vi "ExSpecDebugAppCamera.vi"() -> ()   [LabVIEW 2010]
uses:
  GlobalSpectHdl.vi
  GlobalCamHandle.vi
  GlobalCamOpen.vi
  GlobalInitializeFlag.vi
  GlobalFramesToStr.vi
  GlobalTimingMode.vi
  GlobalAcquireFocusFlag.vi
  GlobalExposure.vi
  GlobalUserBin.vi
  GlobalCenter.vi
  GlobalFullBin.vi
  GlobalReverseFlag.vi
  GlobalIBackImgHndl.vi
  GlobalIFlatImgHndl.vi
panel:
  out "Spectrometer\n active":bool
  out "Camera Opened":bool
  in  "Exit program":bool
  out "error out":errorcluster
  in  "error in (no error)":errorcluster
  in  "Tab Control":T1(tab)
  in  "Focus/Acquire Mode":u32=1 min=1 max=5 step=1
  in  "Number of Frames to store":u32=1 min=1 step=1
  in  "Intensifier":bool
  in  "Readout Port":i32=-1 min=-1 step=1
  in  "ADC Offset 2":i32=-1 min=-1 step=1
  in  "ADC Gain 2":i32=-1 min=-1 step=1
  in  "ADC speed":i32=-2 min=-3 step=1
  in  "Trigger Edge":u32(ring)=1 items=["N/A", "Positive (leading) edge", "Negative (falling) edge"]
  in  "Timing Mode":u32(ring)=1 items=["N/A", "Free Run/Timed", "Trigger First (PM only)", "Ext Sync/Strobed ", "Variable Exp (PM only)", "Flash Mode (PM only)"]
  out "Pixel Time":i32
  out "Bit Depth":i32
  out "ReadOut port":i32
  out "ADC Offset":i32
  out "ADC Gain":i32
  out "ADC Speed":i32
  in  "Set Experiment \nParameters, Initialize \nCamera/Controller":bool
  out "temperature":dbl format="%.2f"
  out "Temperature Read":dbl(slide) scale=-120.0..20.0
  in  "Temperature":dbl format="%.2f"
  in  "Exposure":dbl format="%.2f"
  out "Controller Initialized":bool
  out "Total":u32
  out "Y dim":u32
  out "X dim":u32
  in  "Y Bin":u32=1 min=1 step=1
  in  "Y Start":u32=1 min=1 step=1
  out "center":bool
  out "User":bool
  out "Full":bool
  in  "center strip Button":bool
  in  "User Defined Button":bool
  in  "Full strip Button":bool
  out "Reverse\nActive":bool
  in  "Image Reverse Button":bool
  out "Flat Field\nActive":bool
  out "Background \nActive":bool
  in  "Frame number to read":u32=1 min=1 step=1
  in  "Flat Button":bool
  in  "Back Button":bool
  in  "Full File Name":path
  in  "FileType":u32=67371008
  in  "Get Spectrometer \nInformation":bool
  in  "Set Spectrometer":bool
  out "Current Speed":dbl format="%.2f"
  out "Current Gratting":u32
  out "Current Wavelength":dbl format="%.2f"
  in  "Grating number":u32=1 min=1 step=1
  in  "Wavelength":dbl format="%.2f"
  out "Focus graph":sgl[](graph)
  out "Reverse\nactive":bool
  out "Flat Field\nactive":bool
  out "background\nactive":bool
  in  "Reverse\nbutton":bool
  in  "Flat Field\nbutton":bool
  in  "Background\nbutton":bool
  in  "stop 2":bool
  in  "Start":bool
  out "Camera initialized":bool
  out "Acquire Graph":sgl[](graph)
  out "Collecting Data":bool
  in  "Full File Name\nfor Acqure":path
  in  "OK Button":bool
  out "camera initialized":bool
  # "Note: In order for any parameters to change and be downloaded the initialize button must be hit."
  # "The following are read \nfrom camera after setting\nvalues to left.\n-1 value means it isn't \nsupported by camera."
  # "For Slowest ADC speed set this to -3\nFor Fastest ADC speed set this to -2\nTo use current ADC speed don't  hook up or use -1\notherwise put speed in as kHz"
  # "To use current gain don't hook up or set to -1"
  # "To use current gain don't hook up or set to -1"
  # "To use current gain don't hook up or set to -1"
  # "Pixels coming back\nfrom Camera"
  # "NOTE: if you are using background subtraction or flat field and you change \nthe ROI there is no checks in this example for this."
  # "File Types:\nSPE = 67371008\nTIF   = 67174400\nPMI  = 67436544"
  # "Browse match pattern is set to *.spe.  Modify this if different file type is needed."
  # "Note: This is an example only, the user has to verify that the x,y dimensions match for \nthe background and flat field files with the ROI. This error checking logic is not in this \nexample."
  # "Instructions:\nMake sure camera/controller has been initialized, led should be on.\nPress start button, display should appear.\nWhen done press stop button, display should disappear.\nOnline buttons only work while collecting data, not before,\nto setup before goto On-Line operations tab."
  # "Online operations, well only work while collecting data."
  # "Don't forget to put in a file name below before starting."
  # "Instructions:\nMake sure the camera/controller has been initialized, the light should be on.\nMake sure to put in a file name with path to save data.\nPress Start button and display well pop up and data well be saved in file."
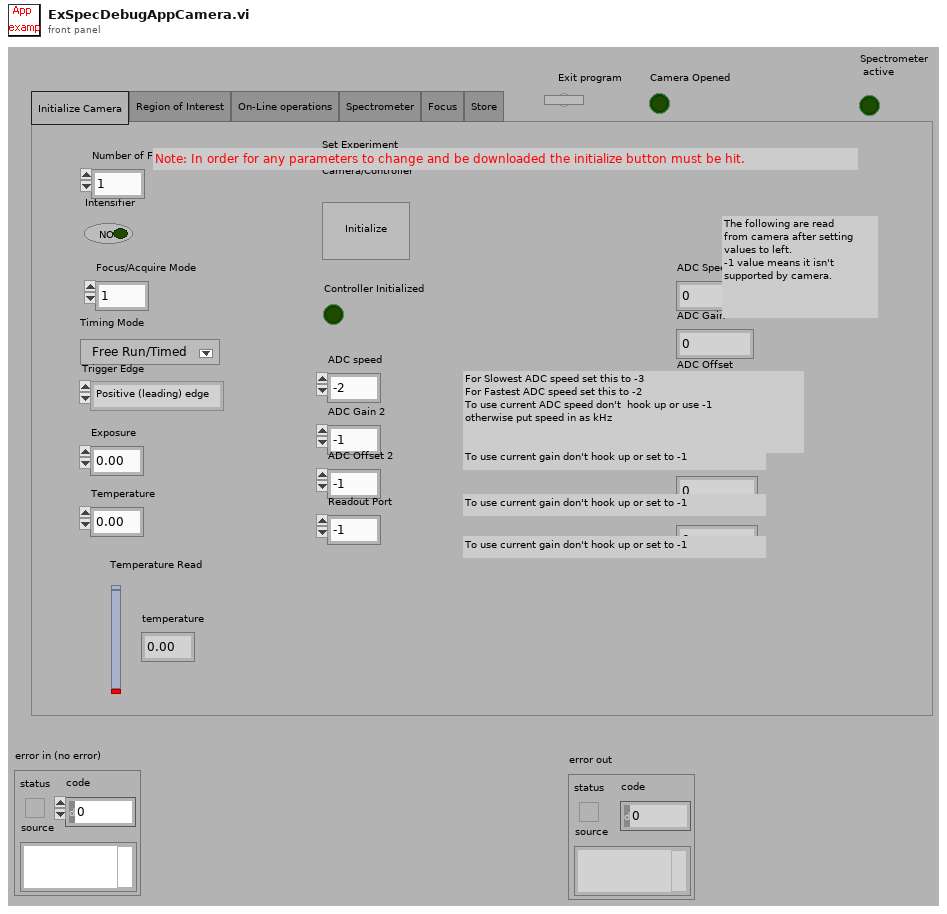
[diagram p1: front panel]
types:
  T1 = enum32{"Initialize Camera", "Region of Interest", "On-Line operations", "Spectrometer", "Focus", "Store"}
  T2 = cluster{"Camera Handle":u32, "Pulser Handle":u32, "File Handle":u32, "Display Handle":u32, "Image Handle":u32}
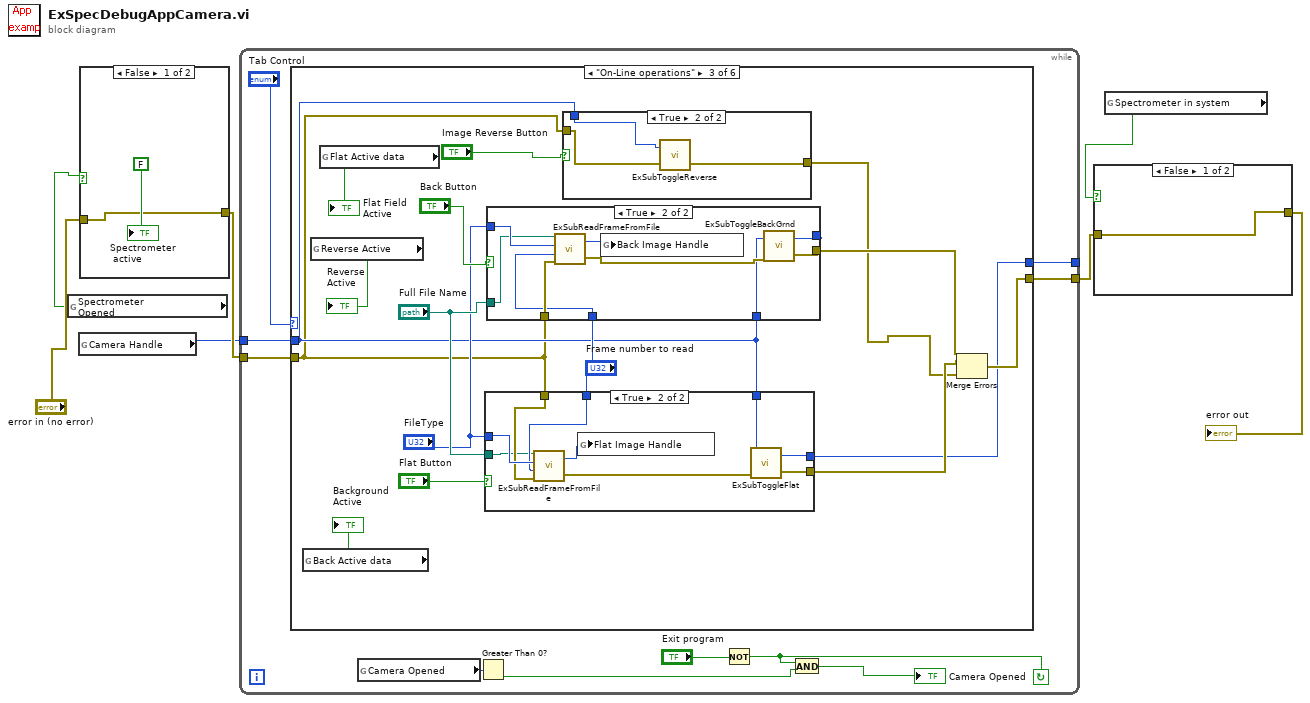
[diagram p0: block diagram]
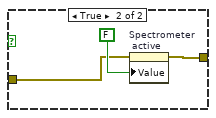
[diagram p2: hidden frame]
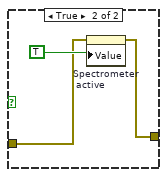
[diagram p3: hidden frame]
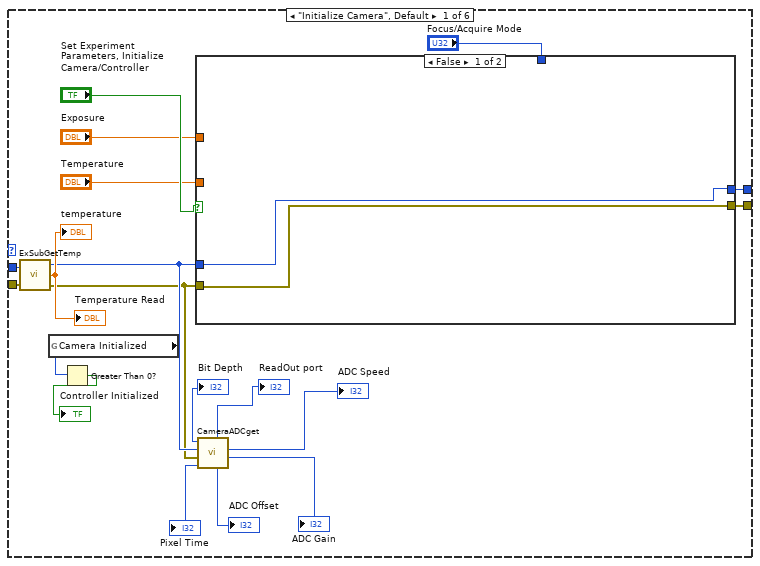
[diagram p4: hidden frame]
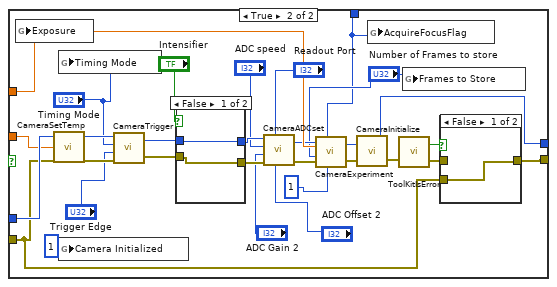
[diagram p5: hidden frame]
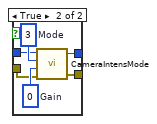
[diagram p7: hidden frame]
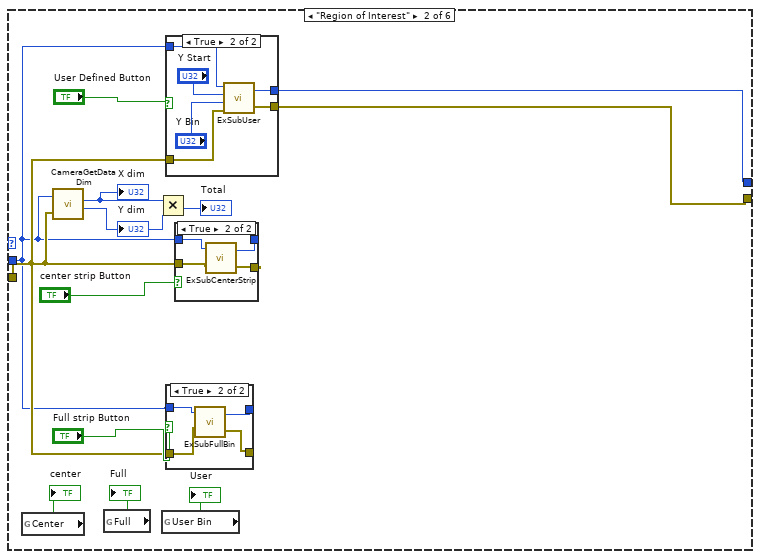
[diagram p8: hidden frame]
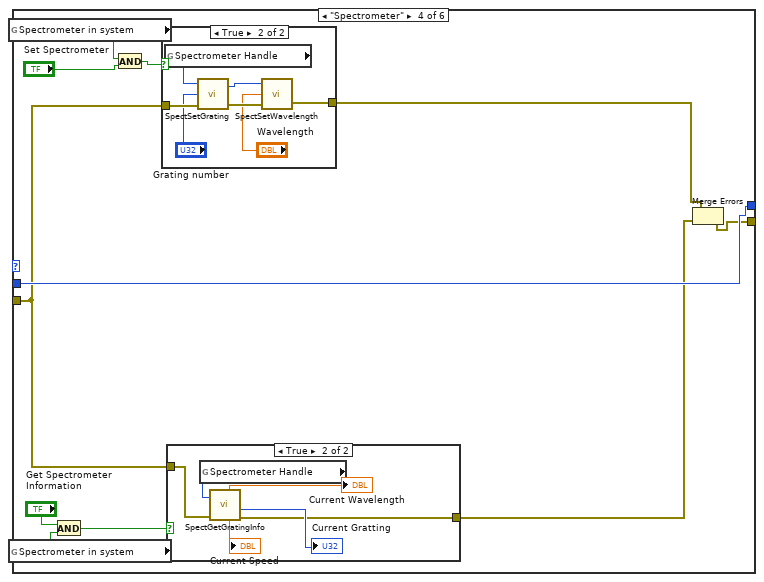
[diagram p15: hidden frame]
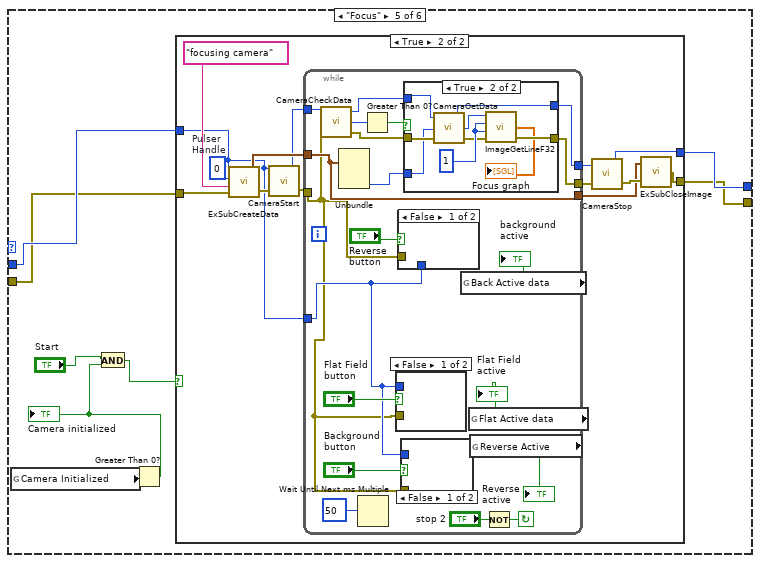
[diagram p18: hidden frame]
diagram:
  n1 = global read "GlobalSpectHdl.vi" "Spectrometer \nOpened"() -> (w1:bool)
  n2 = global read "GlobalCamHandle.vi" "Camera Handle"() -> (w3:u32)
  n3 = case shown="False" w1 {
    tunnel: "error in (no error)" -> [w8 w10]
    tunnel: [w8 w11] -> w4
    frame False {
      "Spectrometer\n active" <- FALSE
    }
    frame True {
      n4 = property on="Spectrometer\n active" class="Bool (strict)"(error in=w10, "Value"=TRUE) -> (error out=w11:errorcluster)  [unwired: 1 in, 1 out]
    }
  }
  n5 = while {
    tunnel: w3 -> [w22]
    tunnel: w4 -> [w19]
    tunnel: [w18] -> _
    tunnel: [w17] -> w6
    stop <- w15 continue-if-true
    n6 = case shown="\"On-Line operations\"" "Tab Control" {
      tunnel: w22 -> [w41 w90 w119 w169 w186 w250]
      tunnel: w19 -> [w33 w91 w118 w162 w185 w249]
      tunnel: [w25 w89 w124 w169 w188 w247] -> w18
      tunnel: [w24 w88 w125 w161 w187 w248] -> w17
      frame "Initialize Camera", Default {
        n7 = call "ExSubGetTemp.vi"("Camera Handle"=w41, "error in (no error)"=w33) -> ("Camera Handle"=w32:u32, "Temperature Real"=→"temperature" →"Temperature Read":dbl, "error out"=w31:errorcluster)
        n8 = global read "GlobalInitializeFlag.vi" "Camera Initialized"() -> (w36:u32)
        n9 = Greater Than 0?(x=w36) -> (x > 0?=→"Controller Initialized":bool)
        n10 = case shown="False" "Set Experiment \nParameters, Initialize \nCamera/Controller" {
          tunnel: "Exposure" -> [_ w62]
          tunnel: "Temperature" -> [_ w71]
          tunnel: w31 -> [w42 w46]
          tunnel: w32 -> [w43 w72]
          tunnel: [w42 w49] -> w24
          tunnel: [w43 w47] -> w25
          tunnel: "Focus/Acquire Mode" -> [_ w44]
          frame False {
          }
          frame True {
            n11 = global write "GlobalExposure.vi" "Exposure"(w62) -> ()
            n12 = call <userlib>:"CameraSetTemp.vi"("error in (no error)"=w46, "Temperature"=w71, "Camera Handle"=w72) -> ("error out"=w61:errorcluster, "Camera Handle"=w60:u32)
            n13 = global write "GlobalTimingMode.vi" "Timing Mode"("Timing Mode") -> ()
            n14 = global write "GlobalInitializeFlag.vi" "Camera Initialized"(1) -> ()
            n15 = call <userlib>:"CameraTrigger.vi"("error in"=w61, "Trigger Edge"="Trigger Edge", "Timing Mode"="Timing Mode", "Camera Handle"=w60) -> ("error out"=w57:errorcluster, "Camera Handle"=w58:u32)
            n16 = case shown="False" "Intensifier" {
              tunnel: [w77 w83] -> w68
              tunnel: [w76 w82] -> w69
              tunnel: w58 -> [w77 w79]
              tunnel: w57 -> [w76 w78]
              frame False {
              }
              frame True {
                w80 = u32 0  # Gain
                w81 = u32 3  # Mode
                n17 = call <userlib>:"CameraIntensMode.vi"("error in"=w78, "Intensifier Gain"=w80, "Mode"=w81, "Camera Handle"=w79) -> ("error out"=w82:errorcluster, "Camera Handle"=w83:u32)
              }
            }
            n18 = call <userlib>:"CameraADCset.vi"("ADC offset"="ADC Offset 2", "Read Out port"="Readout Port", "error in (no error)"=w69, "ADC Gain"="ADC Gain 2", "ADC Speed"="ADC speed", "Camera Handle"=w68) -> ("error out"=w55:errorcluster, "Camera Handle"=w54:u32)
            n19 = call <userlib>:"CameraExperiment.vi"("Number of Accumulations"=1, "Acquire / Focus Flag"=w44, "error in"=w55, "Number of Images"="Number of Frames to store", "Exposure (sec)"=w62, "Camera Handle"=w54) -> ("error out"=w53:errorcluster, "Camera Handle"=w52:u32)
            n20 = call <userlib>:"CameraInitialize.vi"("error in"=w53, "Camera Handle"=w52) -> ("error out"=w48:errorcluster, "Camera Handle"=w47:u32)
            n21 = global write "GlobalAcquireFocusFlag.vi" "AcquireFocusFlag"(w44) -> ()
            n22 = call <userlib>:"ToolKitIsError.vi"("error in"=w48) -> ("error out"=w50:errorcluster, "Error Flag"=w51:bool)  [unwired: 1 in]
            n23 = global write "GlobalFramesToStr.vi" "Frames to Store"("Number of Frames to store") -> ()
            n24 = case shown="False" w51 {
              tunnel: w50 -> [_ w75]
              tunnel: [w74 w75] -> w49
              tunnel: w46 -> [w74 _]
              frame False {
              }
              frame True {
              }
            }
          }
        }
        n25 = call <userlib>:"CameraADCget.vi"("Camera handle"=w32, "error in (no error)"=w31) -> ("Bit Depth"=→"Bit Depth":i32, "Pixel Time"=→"Pixel Time":i32, "Readout Port"=→"ReadOut port":i32, "ADC Offset"=→"ADC Offset":i32, "ADC Speed"=→"ADC Speed":i32, "ADC Gain"=→"ADC Gain":i32)  [unwired: 2 out]
      }
      frame "Region of Interest" {
        n26 = global read "GlobalCenter.vi" "Center"() -> (→"center":bool)
        n27 = call <userlib>:"CameraGetDataDim.vi"("Camera Handle"=w90, "error in"=w91) -> ("Xdim"=w87:u32, "Ydim"=w86:u32)  [unwired: 2 out]
        "X dim" <- w87
        "Y dim" <- w86
        n28 = global read "GlobalFullBin.vi" "Full"() -> (→"Full":bool)
        n29 = Multiply(x=w87, y=w86) -> (x*y=→"Total":u32)
        n30 = global read "GlobalUserBin.vi" "User Bin"() -> (→"User":bool)
        n31 = case shown="True" "User Defined Button" {
          tunnel: w90 -> [w109 w116]
          tunnel: [w109 w111] -> w89
          tunnel: w91 -> [w110 w113]
          tunnel: [w110 w112] -> w88
          frame False {
          }
          frame True {
            n32 = call "ExSubUser.vi"("error in (no error)"=w113, "Y Bin"="Y Bin", "Y Start"="Y Start", "Camera Handle"=w116) -> ("error out"=w112:errorcluster, "Camera Handle"=w111:u32)
          }
        }
        n33 = case shown="True" "Full strip Button" {
          tunnel: w90 -> [w98 w102]
          tunnel: [w98 w100] -> _
          tunnel: w91 -> [w97 w101]
          tunnel: [w97 w99] -> _
          frame False {
          }
          frame True {
            n34 = call "ExSubFullBin.vi"("error in (no error)"=w101, "Camera Handle"=w102) -> ("error out"=w99:errorcluster, "Camera Handle"=w100:u32)
          }
        }
        n35 = case shown="True" "center strip Button" {
          tunnel: w90 -> [w104 w107]
          tunnel: [w104 w106] -> _
          tunnel: w91 -> [w103 w108]
          tunnel: [w103 w105] -> _
          frame False {
          }
          frame True {
            n36 = call "ExSubCenterStrip.vi"("error in (no error)"=w108, "Camera Handle"=w107) -> ("error out"=w105:errorcluster, "Camera Handle"=w106:u32)
          }
        }
      }
      frame "On-Line operations" {
        n37 = global read "GlobalIBackImgHndl.vi" "Back Active data"() -> (→"Background \nActive":bool)
        n38 = global read "GlobalReverseFlag.vi" "Reverse Active"() -> (→"Reverse\nActive":bool)
        n39 = global read "GlobalIFlatImgHndl.vi" "Flat Active data"() -> (→"Flat Field\nActive":bool)
        n40 = case shown="True" "Flat Button" {
          tunnel: "Full File Name" -> [_ w144]
          tunnel: "FileType" -> [_ w147]
          tunnel: w118 -> [w138 w145]
          tunnel: [w138 w140] -> w126
          tunnel: "Frame number to read" -> [_ w146]
          tunnel: w119 -> [w137 w142]
          tunnel: [w137 w141] -> w124
          frame False {
          }
          frame True {
            n41 = call "ExSubReadFrameFromFile.vi"("error in (no error)"=w145, "Frame to pull off"=w146, "File type"=w147, "path to file to open"=w144) -> ("error out"=w139:errorcluster, "Image Handle"=w143:u32)
            n42 = global write "GlobalIFlatImgHndl.vi" "Flat Image Handle"(w143) -> ()
            n43 = call "ExSubToggleFlat.vi"("error in (no error)"=w139, "Camera Handle"=w142) -> ("error out"=w140:errorcluster, "Camera Handle"=w141:u32)
          }
        }
        n44 = case shown="True" "Back Button" {
          tunnel: "Full File Name" -> [_ w156]
          tunnel: "FileType" -> [_ w157]
          tunnel: w118 -> [w149 w158]
          tunnel: [w149 w152] -> w127
          tunnel: "Frame number to read" -> [_ w155]
          tunnel: w119 -> [w148 w151]
          tunnel: [w148 w150] -> _
          frame False {
          }
          frame True {
            n45 = call "ExSubReadFrameFromFile.vi"("error in (no error)"=w158, "Frame to pull off"=w155, "File type"=w157, "path to file to open"=w156) -> ("error out"=w153:errorcluster, "Image Handle"=w154:u32)
            n46 = global write "GlobalIBackImgHndl.vi" "Back Image Handle"(w154) -> ()
            n47 = call "ExSubToggleBackGrnd.vi"("error in (no error)"=w153, "Camera Handle"=w151) -> ("error out"=w152:errorcluster, "Camera Handle"=w150:u32)
          }
        }
        n48 = case shown="True" "Image Reverse Button" {
          tunnel: w119 -> [_ w135]
          tunnel: w118 -> [w133 w136]
          tunnel: [w133 w134] -> w117
          frame False {
          }
          frame True {
            n49 = call "ExSubToggleReverse.vi"("error in (no error)"=w136, "Camera Handle"=w135) -> ("error out"=w134:errorcluster)  [unwired: 1 out]
          }
        }
        n50 = Merge Errors(w127, w126, w117) -> (w125:errorcluster)
      }
      frame "Spectrometer" {
        n51 = global read "GlobalSpectHdl.vi" "Spectrometer in system"() -> (w168:bool)
        n52 = global read "GlobalSpectHdl.vi" "Spectrometer in system"() -> (w165:bool)
        n53 = And(x="Get Spectrometer \nInformation", y=w165) -> (x .and. y?=w163:bool)
        n54 = And(x=w168, y="Set Spectrometer") -> (x .and. y?=w166:bool)
        n55 = case shown="True" w166 {
          tunnel: w162 -> [w177 w183]
          tunnel: [w177 w178] -> w159
          frame False {
          }
          frame True {
            n56 = global read "GlobalSpectHdl.vi" "Spectrometer Handle"() -> (w184:u32)
            n57 = call <userlib>:"SpectSetGrating.vi"("error in"=w183, "Grating Number"="Grating number", "Sepctrometer Handle"=w184) -> ("error out"=w180:errorcluster, "Spectrometer Handle"=w181:u32)
            n58 = call <userlib>:"SpectSetWavelength.vi"("error in"=w180, "Wavelength"="Wavelength", "Spectrometer Handle"=w181) -> ("error out"=w178:errorcluster)  [unwired: 1 out]
          }
        }
        n59 = case shown="True" w163 {
          tunnel: w162 -> [w170 w175]
          tunnel: [w170 w172] -> w160
          frame False {
          }
          frame True {
            n60 = global read "GlobalSpectHdl.vi" "Spectrometer Handle"() -> (w176:u32)
            n61 = call <userlib>:"SpectGetGratingInfo.vi"("Spectrometer Handle"=w176, "error in"=w175) -> ("Current Wavelength"=→"Current Wavelength":dbl, "Current Speed"=→"Current Speed":dbl, "Current Grating"=→"Current Gratting":i16, "error out"=w172:errorcluster)  [unwired: 2 out]
          }
        }
        n62 = Merge Errors(w159, w160) -> (w161:errorcluster)
      }
      frame "Focus" {
        n63 = global read "GlobalInitializeFlag.vi" "Camera Initialized"() -> (w190:u32)
        n64 = Greater Than 0?(x=w190) -> (x > 0?=w189:bool)
        "Camera initialized" <- w189
        n65 = And(x="Start", y=w189) -> (x .and. y?=w192:bool)
        n66 = case shown="True" w192 {
          tunnel: w185 -> [w193 w204]
          tunnel: w186 -> [w194 w197]
          tunnel: [w194 w202] -> w188
          tunnel: [w193 w201] -> w187
          frame False {
          }
          frame True {
            w205 = u32 0  # Pulser  Handle
            n67 = call "ExSubCreateData.vi"("error in (no error)"=w204, "File and Display Name"="focusing camera", "Pulser Handle"=w205, "Camera Handle"=w197) -> ("error out"=w206:errorcluster, "Handles Out"=w208:T2)
            n68 = call <userlib>:"CameraStart.vi"("error in"=w206, "Camera Handle"=w197) -> ("error out"=w207:errorcluster, "Camera Handle"=w199:u32)
            n69 = while {
              tunnel: w208 -> [w210]
              tunnel: w207 -> [w209]
              tunnel: w197 -> [w222]
              tunnel: w199 -> [w214]
              tunnel: [w213] -> w198
              tunnel: [w212] -> w196
              tunnel: [w210] -> w195
              stop <- w226 continue-if-true
              n70 = call <userlib>:"CameraCheckData.vi"("Camera Handle"=w214, "error in"=w209) -> ("Camera Handle"=w216:u32, "Number Of Frames Available"=w218:i32, "error out"=w215:errorcluster)
              n71 = Unbundle(w210) -> ("Image Handle"=w211:u32)  [unwired: 4 out]
              n72 = Wait Until Next ms Multiple(millisecond multiple=u32 50) -> ()  [unwired: 1 out]
              n73 = Greater Than 0?(x=w218) -> (x > 0?=w217:bool)
              n74 = case shown="False" "Flat Field\nbutton" {
                tunnel: w222 -> [_ w242]
                tunnel: w209 -> [_ w243]
                frame False {
                }
                frame True {
                  n75 = call "ExSubToggleFlat.vi"("error in (no error)"=w243, "Camera Handle"=w242) -> ()  [unwired: 2 out]
                }
              }
              n76 = case shown="False" "Reverse\nbutton" {
                tunnel: w209 -> [_ w245]
                tunnel: w222 -> [_ w244]
                frame False {
                }
                frame True {
                  n77 = call "ExSubToggleReverse.vi"("error in (no error)"=w245, "Camera Handle"=w244) -> ()  [unwired: 2 out]
                }
              }
              n78 = case shown="False" "Background\nbutton" {
                tunnel: w222 -> [_ w241]
                tunnel: w209 -> [_ w240]
                frame False {
                }
                frame True {
                  n79 = call "ExSubToggleBackGrnd.vi"("error in (no error)"=w240, "Camera Handle"=w241) -> ()  [unwired: 2 out]
                }
              }
              n80 = case shown="True" w217 {
                tunnel: w216 -> [w230 w239]
                tunnel: w215 -> [w229 w238]
                tunnel: [w229 w233] -> w212
                tunnel: [w230 w232] -> w213
                tunnel: w211 -> [_ w237]
                frame False {
                }
                frame True {
                  w235 = 1
                  n81 = call <userlib>:"CameraGetData.vi"("error in"=w238, "Data Handle"=w237, "Camera Handle"=w239) -> ("error out"=w234:errorcluster, "Data Handle"=w236:u32, "Camera Handle"=w232:u32)
                  n82 = call <userlib>:"ImageGetLineF32.vi"("error in"=w234, "Z Position"=w235, "Y Position"=w235, "Data Handle"=w236) -> ("error out"=w233:errorcluster, "Array F32"=→"Focus graph":sgl[])  [unwired: 1 out]
                }
              }
              n83 = global read "GlobalIBackImgHndl.vi" "Back Active data"() -> (→"background\nactive":bool)
              n84 = global read "GlobalIFlatImgHndl.vi" "Flat Active data"() -> (→"Flat Field\nactive":bool)
              n85 = global read "GlobalReverseFlag.vi" "Reverse Active"() -> (→"Reverse\nactive":bool)
              n86 = Not(x="stop 2") -> (.not. x?=w226:bool)
            }
            n87 = call <userlib>:"CameraStop.vi"("error in"=w196, "Camera Handle"=w198) -> ("error out"=w203:errorcluster, "Camera Handle"=w202:u32)
            n88 = call "ExSubCloseImage.vi"("error in (no error)"=w203, "Handles In"=w195) -> ("error out"=w201:errorcluster)
          }
        }
      }
      frame "Store" {
        n89 = global read "GlobalInitializeFlag.vi" "Camera Initialized"() -> (w252:u32)
        n90 = Greater Than 0?(x=w252) -> (x > 0?=w251:bool)
        "camera initialized" <- w251
        n91 = And(x="OK Button", y=w251) -> (x .and. y?=w254:bool)
        n92 = case shown="True" w254 {
          tunnel: w250 -> [w256 w260]
          tunnel: w249 -> [w255 w264]
          tunnel: [w255 w265] -> w248
          tunnel: [w256 w261] -> w247
          frame False {
          }
          frame True {
            w271 = u32 0  # Pulser Handle
            n93 = global read "GlobalFramesToStr.vi" "Frames to Store"() -> (w267:u32)
            n94 = property on="Collecting Data" class="Bool (strict)"(error in=w264, "Value"=TRUE) -> (error out=w263:errorcluster)  [unwired: 1 in, 1 out]
            n95 = Path To String(path="Full File Name\nfor Acqure") -> (string=w269:string)
            n96 = call "ExSubCreateFile.vi"("error in (no error)"=w263, "File and Display Name"=w269, "Pulser Handle"=w271, "Camera Handle"=w260) -> ("error out"=w272:errorcluster, "Handles Out"=w257:T2)
            n97 = call <userlib>:"CameraStart.vi"("error in"=w272, "Camera Handle"=w260) -> ("error out"=w259:errorcluster, "Camera Handle"=w266:u32)
            n98 = for {
              N: w267 -> [_]
              tunnel: w260 -> [w275]
              tunnel: w259 -> [w274]
              tunnel: [w273] -> w258
              n99 = while {
                tunnel: [w280] -> w273
                tunnel: w275 -> [w278]
                tunnel: w274 -> [w277]
                stop <- w281 stop-if-true
                n100 = call <userlib>:"CameraCheckData.vi"("Camera Handle"=w278, "error in"=w277) -> ("Camera Handle"=w283:u32, "Number Of Frames Available"=w285:i32, "error out"=w282:errorcluster)
                n101 = Greater Than 0?(x=w285) -> (x > 0?=w284:bool)
                n102 = case shown="True" w284 {
                  selector: w284 -> [w286 w294]
                  tunnel: w283 -> [_ w296]
                  tunnel: w282 -> [w287 w295]
                  tunnel: [w286 w294] -> w281
                  tunnel: [w287 w289] -> w280
                  frame False {
                  }
                  frame True {
                    w290 = 1
                    n103 = call <userlib>:"CameraGetData.vi"("error in"=w295, "Camera Handle"=w296) -> ("error out"=w293:errorcluster, "Data Handle"=w291:u32)  [unwired: 1 in, 1 out]
                    n104 = call <userlib>:"FileSaveData.vi"("error in"=w293, "Image Handle"=w291) -> ("error out"=w292:errorcluster)  [unwired: 1 in, 1 out]
                    n105 = call <userlib>:"ImageGetLineF32.vi"("error in"=w292, "Z Position"=w290, "Y Position"=w290, "Data Handle"=w291) -> ("error out"=w289:errorcluster, "Array F32"=→"Acquire Graph":sgl[])  [unwired: 1 out]
                  }
                }
                n106 = Wait Until Next ms Multiple(millisecond multiple=u32 50) -> ()  [unwired: 1 out]
              }
              n107 = Wait Until Next ms Multiple(millisecond multiple=u32 50) -> ()  [unwired: 1 out]
            }
            n108 = call <userlib>:"CameraStop.vi"("error in"=w258, "Camera Handle"=w266) -> ("error out"=w268:errorcluster, "Camera Handle"=w261:u32)
            n109 = call "ExSubCloseFileImage.vi"("error in (no error)"=w268, "Handles In"=w257) -> ("error out"=w265:errorcluster)
          }
        }
        "Collecting Data" <- FALSE
      }
    }
    n110 = global read "GlobalCamOpen.vi" "Camera Opened"() -> (w16:u32)
    n111 = Greater Than 0?(x=w16) -> (x > 0?=w14:bool)
    n112 = Not(x="Exit program") -> (.not. x?=w15:bool)
    n113 = And(x=w15, y=w14) -> (x .and. y?=→"Camera Opened":bool)
  }
  n114 = global read "GlobalSpectHdl.vi" "Spectrometer in system"() -> (w5:bool)
  n115 = case shown="False" w5 {
    tunnel: w6 -> [w297 w298]
    tunnel: [w297 w300] -> w7
    frame False {
    }
    frame True {
      n116 = property on="Spectrometer\n active" class="Bool (strict)"(error in=w298, "Value"=FALSE) -> (error out=w300:errorcluster)  [unwired: 1 in, 1 out]
    }
  }
  "error out" <- w7
